vi "Get Measurements.vi"(8 "error in (no error)":errorcluster) -> (0 "error out":errorcluster, 3 "measurements":T1[](array[typedef]))   [LabVIEW 2023]
uses:
  builds/PowerModuleInterface/PowerModuleInterface PPL/PowerModuleInterface.lvlibp/Classes/PowerModule_interface/PowerModuleInterface.lvclass
  builds/PowerModuleInterface/PowerModuleInterface PPL/PowerModuleInterface.lvlibp/Classes/PowerModule_interface/Measurements.ctl
panel:
  in  "Power Module":refnum<class "PowerModuleInterface.lvclass">
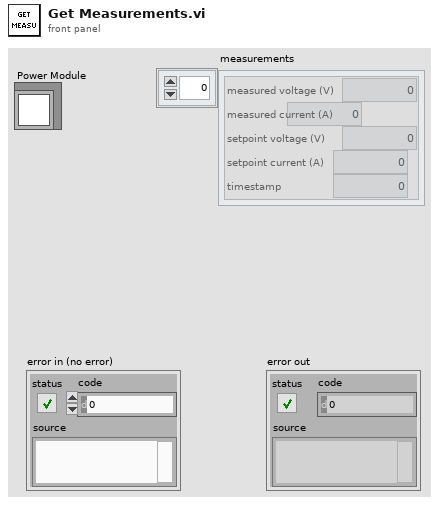
[diagram p1: front panel]
types:
  T1 = typedef "PowerModuleInterface.lvlibp/PowerModuleInterface.lvclass/Measurements.ctl" = cluster{"measured voltage (V)":dbl, "measured current (A)":dbl, "setpoint voltage (V)":dbl, "setpoint current (A)":dbl, "timestamp":dbl}
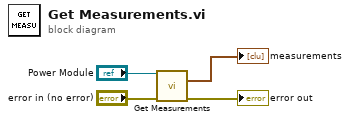
[diagram p0: block diagram]
diagram:
  n1 = call-dynamic "Get Measurements.vi"("object in"="Power Module", "Error In"="error in (no error)") -> ("measurements"=→"measurements":T1[], "Error Out"=→"error out":errorcluster)  [unwired: 11 in, 1 out]
